vi "for axis(360) (SubVI).vi"(1 "angle":ext) -> (0 "axis":ext)   [LabVIEW 2017]
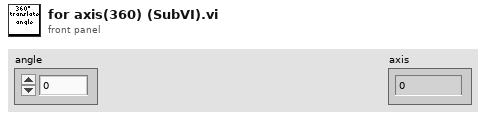
[diagram p1: front panel]
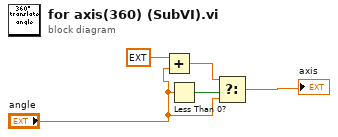
[diagram p0: block diagram]
diagram:
  n1 = Add(x=ext 360.0, y="angle") -> (x+y=w2:ext)
  n2 = Less Than 0?(x="angle") -> (x < 0?=w4:bool)
  n3 = Select(t=w2, s=w4, f="angle") -> (s? t:f=→"axis":ext)
